vi "CAN_testing.vi"() -> ()   [LabVIEW 2017]
doc: "Demonstrates how to write and receive CAN frames via the Network Interface on the same port. \n\nTo write and receive frames via the Network Interface:\n- select the CAN Network Interface (i.e. CAN0, CAN1, etc.)\n- select the Baud Rate\n- run the VI\n- press the write button to write frames to the can bus\n\nEnable RTR Button to send a Remote Transmission Request or to simply send an empty Frame to request an Answer Frame from a connected device.\n\nEnable Extended Button to write extended Identifier Format. This is done by setting the 30th bit to enable extended format with the driver."
uses:
  <vilib>/nican/nican.llb/CanFrameTimed.ctl
  <vilib>/nican/nican.llb/ncNetAttr.ctl
panel:
  out "ActualDataSize (Frames)":u32
  out "Data":T1[](array[typedef]) {"Data" format="%.0x"; "ArbitrationId" format="%.0x"; "Timestamp" format="%<%I:%M:%S%3u %p\n%m/%d/%Y>T"}
  in  "IND2":bool
  in  "IND1":bool
  in  "interface":string(combo)="CAN0" caption="Interface"
  in  "shutdown":bool
  # "PRESS AND HOLD"
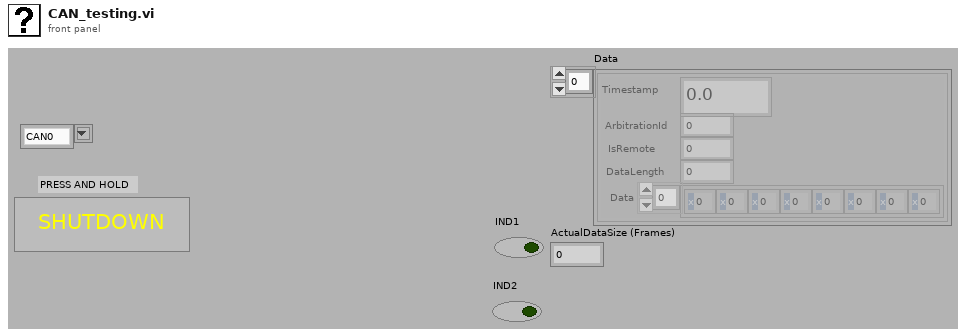
[diagram p1: front panel]
types:
  T1 = typedef "CanFrameTimed.ctl" = cluster{"Timestamp":dbl, "ArbitrationId":u32, "IsRemote":u8, "DataLength":u8, "Data":u8[]}
  T2 = typedef "ncNetAttr.ctl" = cluster{"Start On Open":enum32{"FALSE", "TRUE"}, "Baud Rate":u32, "Read Queue Length":u32, "Write Queue Length":u32, "Standard Comparator":u32, "Standard Mask":u32, "Extended Comparator":u32, "Extended Mask":u32}
  T3 = typedef "xobjhandle.ctl" = u32
  T4 = cluster{dbl, u32, "IsRemote":u8, "DataLength":u8, u8[]}
  T5 = cluster{dbl, u32, "IsRemote":u8, "DataLength":u8, u8[]}[]
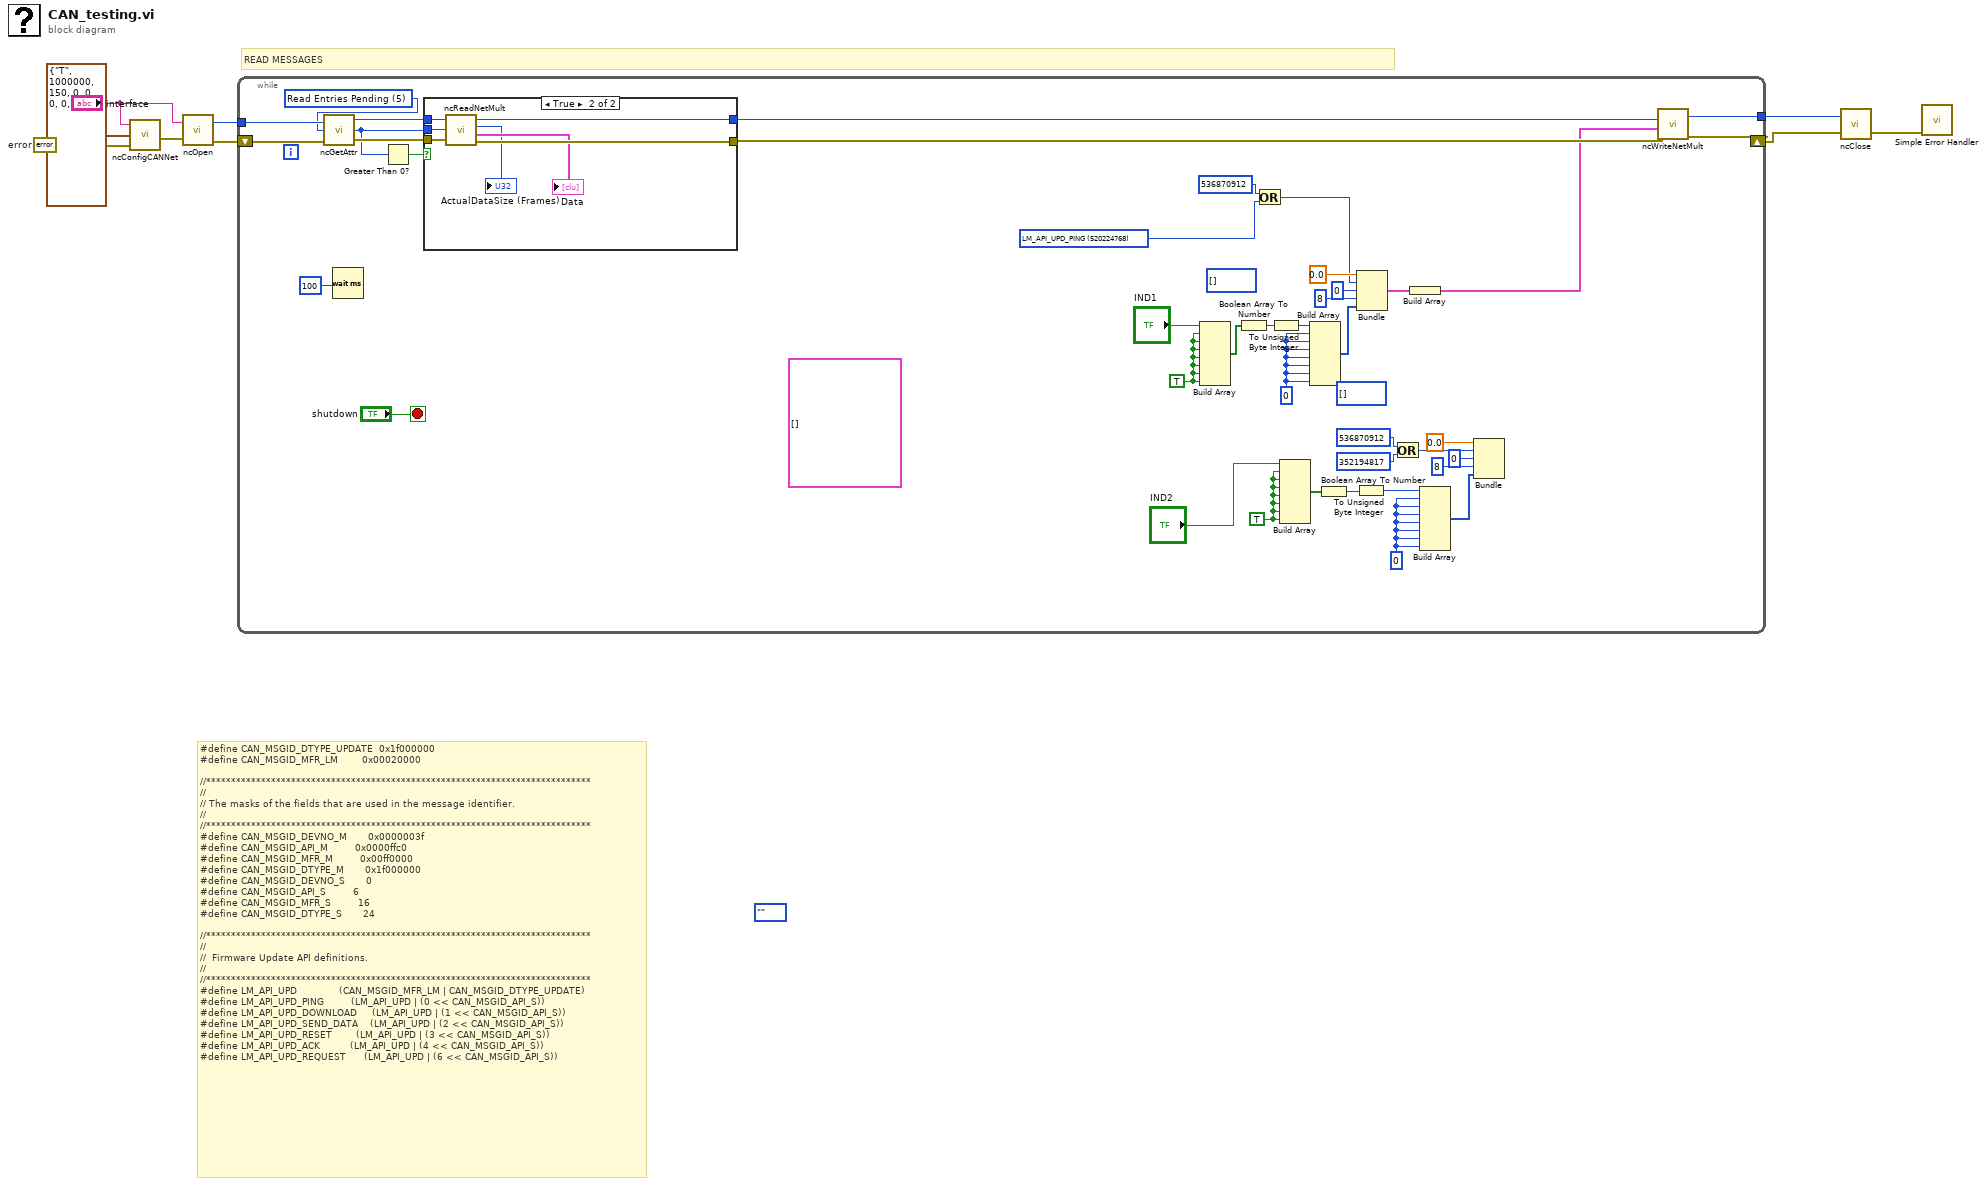
[diagram p0: block diagram]
diagram:
  (unwired) enum32{""}.""
  w5 = errorcluster {"status"=FALSE, "code"=0, "source"=""}  # error
  # "#define CAN_MSGID_DTYPE_UPDATE  0x1f000000\n#define CAN_MSGID_MFR_LM        0x00020000\n\n//*****************************************************************************\n//\n// The masks of the fields that are used in the message identifier.\n//\n//*****************************************************************************\n#define CAN_MSGID_DEVNO_M       0x0000003f\n#define CAN_MSGID_API_M         0x0000ffc0\n#define CAN_MSGID_MFR_M         0x00ff0000\n#define CAN_MSGID_DTYPE_M       0x1f000000\n#define CAN_MSGID_DEVNO_S       0\n#define CAN_MSGID_API_S         6\n#define CAN_MSGID_MFR_S         16\n#define CAN_MSGID_DTYPE_S       24\n\n//*****************************************************************************\n//\n//  Firmware Update API definitions.\n//\n//*****************************************************************************\n#define LM_API_UPD              (CAN_MSGID_MFR_LM | CAN_MSGID_DTYPE_UPDATE)\n#define LM_API_UPD_PING         (LM_API_UPD | (0 << CAN_MSGID_API_S))\n#define LM_API_UPD_DOWNLOAD     (LM_API_UPD | (1 << CAN_MSGID_API_S))\n#define LM_API_UPD_SEND_DATA    (LM_API_UPD | (2 << CAN_MSGID_API_S))\n#define LM_API_UPD_RESET        (LM_API_UPD | (3 << CAN_MSGID_API_S))\n#define LM_API_UPD_ACK          (LM_API_UPD | (4 << CAN_MSGID_API_S))\n#define LM_API_UPD_REQUEST      (LM_API_UPD | (6 << CAN_MSGID_API_S))"
  # "READ MESSAGES"
  n1 = call <vilib>:"ncConfigCANNet.vi"("Error in"=w5, "CAN Network Interface Config"=T2 {"Start On Open"=enum."TRUE", "Baud Rate"=1000000, "Read Queue Length"=150, "Write Queue Length"=0, "Standard Comparator"=0, "Standard Mask"=0, "Extended Comparator"=0, "Extended Mask"=0}, "ObjName"="interface") -> ("Error out"=w6:errorcluster)  [unwired: 2 in]
  n2 = call <vilib>:"ncOpen.vi"("Error in"=w6, "ObjName"="interface") -> ("Error out"=w9:errorcluster, "ObjHandle out"=w7:T3)
  n3 = while {
    tunnel: w7 -> [w44]
    tunnel: [w49] -> w2
    shift-right: [w50] -> w1
    shift-left: w9 -> [w43]
    stop <- "shutdown" stop-if-true
    (unwired) u8[] [] ("appended array")
    w11 = u32 520224768 items=["LM_API_UPD_PING"=520224768, "LM_API_UPD_DOWNLOAD"=520224780, "LM_API_UPD_SEND_DATA"=520224792, "LM_API_UPD_RESET"=520224960, "LM_API_UPD_ACK"=520224864, "LM_API_UPD_REQUEST"=520227516]
    (unwired) u8[] [] ("appended array")
    (unwired) T1[] [] ("Data")
    w21 = TRUE ("element")
    w23 = TRUE ("element")
    w26 = u8 0
    w30 = u8 0
    w40 = u32 5 items=["(reserved)", "Protocol Version", "Software Version", "Object State", "(reserved)", "Read Entries Pending", "Write Entries Pending", "ReadMult Size for Notification", "Listen Only?", "Self Reception?", "Transmit Error Counter", "Receive Error Counter", "Single Shot Transmit?", "Series 2 Filter Mode", "Series 2 Mask", "Series 2 Comparator", "Serial Number", "Form Factor", "Series", "Transceiver Type", "Interface Number", "Series 2 Error/Arb Capture", "Transceiver Mode", "Transceiver External Outputs", "Transceiver External Inputs", "Start Trigger Behavior", "Log Comm Warnings", "User RTSI Frame", "Transmit Mode", "Log Start Trigger?", "Timestamp Format", "Master Timebase Rate", "Virtual Bus Timing"] ("AttrId")
    n4 = call <vilib>:"ncGetAttr.vi"("Error in"=w43, "AttrId"=w40, "ObjHandle in"=w44) -> ("Error out"=w48:errorcluster, "AttrValue"=w45:u32, "ObjHandle out"=w47:T3)
    n5 = Wait (ms)(milliseconds to wait=u32 100 ("millisecond multiple")) -> ()  [unwired: 1 out]
    n6 = Greater Than 0?(x=w45) -> (x > 0?=w46:bool)
    n7 = case shown="True" w46 {
      tunnel: [w51 w59] -> w41
      tunnel: [w52 w58] -> w42
      tunnel: w45 -> [_ w57]
      tunnel: w48 -> [w51 w56]
      tunnel: w47 -> [w52 w55]
      frame False {
      }
      frame True {
        n8 = call <vilib>:"ncReadNetMult.vi"("ObjHandle in"=w55, "Requested Number of Frames"=w57, "Error in"=w56) -> ("ObjHandle out"=w58:T3, "ActualDataSize (Frames)"=→"ActualDataSize (Frames)":u32, "Data"=→"Data":T1[], "Error out"=w59:errorcluster)
      }
    }
    n9 = Build Array("IND1", w23, w23, w23, w23, w23, w23, w23) -> (w17:bool[])
    n10 = Boolean Array To Number(Boolean array=w17) -> (number=w19:u32)
    n11 = Or(x=u32 536870912 ("y"), y=w11) -> (x .or. y?=w12:u32)
    n12 = To Unsigned Byte Integer(number=w19) -> (unsigned 8bit integer=w18:u8)
    n13 = Build Array("IND2", w21, w21, w21, w21, w21, w21, w21) -> (w22:bool[])
    n14 = Build Array(w18, w26, w26, w26, w26, w26, w26, w26) -> (w10:u8[])
    n15 = Boolean Array To Number(Boolean array=w22) -> (number=w15:u32)
    n16 = To Unsigned Byte Integer(number=w15) -> (unsigned 8bit integer=w16:u8)
    n17 = Bundle(0.0, w12, "IsRemote"=u8 0, "DataLength"=u8 8, w10) -> (w25:T4)  [unwired: 1 in]
    n18 = Or(x=u32 536870912 ("y"), y=u32 352194817) -> (x .or. y?=w36:u32)
    n19 = Build Array(w25) -> (w14:T5)
    n20 = Build Array(w16, w30, w30, w30, w30, w30, w30, w30) -> (w32:u8[])
    n21 = Bundle(0.0, w36, "IsRemote"=u8 0, "DataLength"=u8 8, w32) -> ()  [unwired: 1 in, 1 out]
    n22 = call <vilib>:"ncWriteNetMult.vi"("Error in"=w41, "Data"=w14, "ObjHandle in"=w42) -> ("Error out"=w50:errorcluster, "ObjHandle out"=w49:T3)  [unwired: 7 in]
  }
  n23 = call <vilib>:"ncClose.vi"("Error in"=w1, "ObjHandle in"=w2) -> ("Error out"=w3:errorcluster)  [unwired: 1 in]
  n24 = call <vilib>:"Simple Error Handler.vi"("error in (no error)"=w3) -> ()  [unwired: 4 in, 5 out]
